vi "detection.vi"() -> (0 "Counts":u32=198)   [LabVIEW 2012]
uses:
  <vilib>/DAQmx/write.llb/DAQmx Write (Digital Wfm 1Chan NSamp).vi
  <vilib>/DAQmx/write.llb/DAQmx Write (Digital 1D Bool 1Chan 1Samp).vi
  <vilib>/DAQmx/read.llb/DAQmx Read (Counter 1D U32 1Chan NSamp).vi
  <vilib>/Waveform/DWDTOps.llb/DWDT Boolean Array to Digital.vi
  <vilib>/DAQmx/create/channels.llb/DAQmx Create Channel (CO-Pulse Generation-Frequency).vi
  <vilib>/DAQmx/configure/timing.llb/DAQmx Timing (Implicit).vi
  <vilib>/DAQmx/create/channels.llb/DAQmx Create Channel (CI-Count Edges).vi
  <vilib>/DAQmx/configure/timing.llb/DAQmx Timing (Sample Clock).vi
  <vilib>/DAQmx/create/channels.llb/DAQmx Create Channel (DO-Digital Output).vi
  <vilib>/Waveform/DWDTOps.llb/DWDT Uncompress Digital.vi
  <vilib>/DAQmx/miscellaneous.llb/DAQmx Fill In Error Info.vi
  <resource>/objmgr/daqmx.rc
panel:
  in  "Use delay":bool
  in  "Final states":bool[](array[boolean])
  in  "Delay (ms)":dbl
  out "data":u32[](graph)=[0, 0, 1, 0, 1, 0, 2, 0, 2, 4, 2, 2, 0, 2, 0, 0, 2, 1, 2, 1]
  out "Output":bool=TRUE
  in  "Threshold":dbl=200.0
  in  "Detection length (ms)":dbl=20.0 min=1.0
  in  "Off times":i32[](array[numeric])=[0, 0, 0, 0, 0, 0, 0, 0]
  in  "On times":i32[](array[numeric])=[0, 0, 0, 0, 0, 0, 0, 0]
  # "Pockel"
  # "LED"
  # "Tsunami"
  # "RF"
  # "Orange"
  # "Blue"
  # "Red"
  # "Times in 0.1 uS"
  # "Use -1 to never switch"
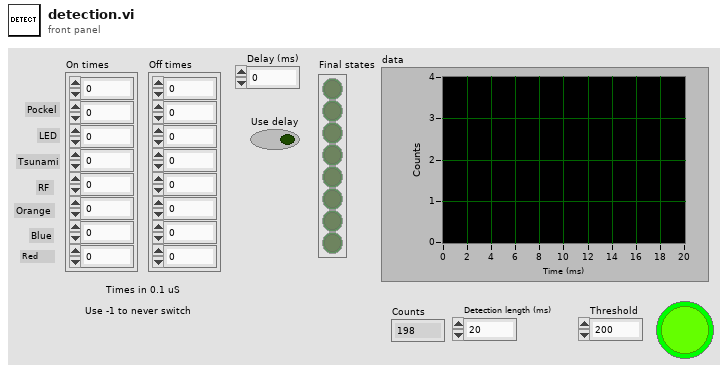
[diagram p1: front panel]
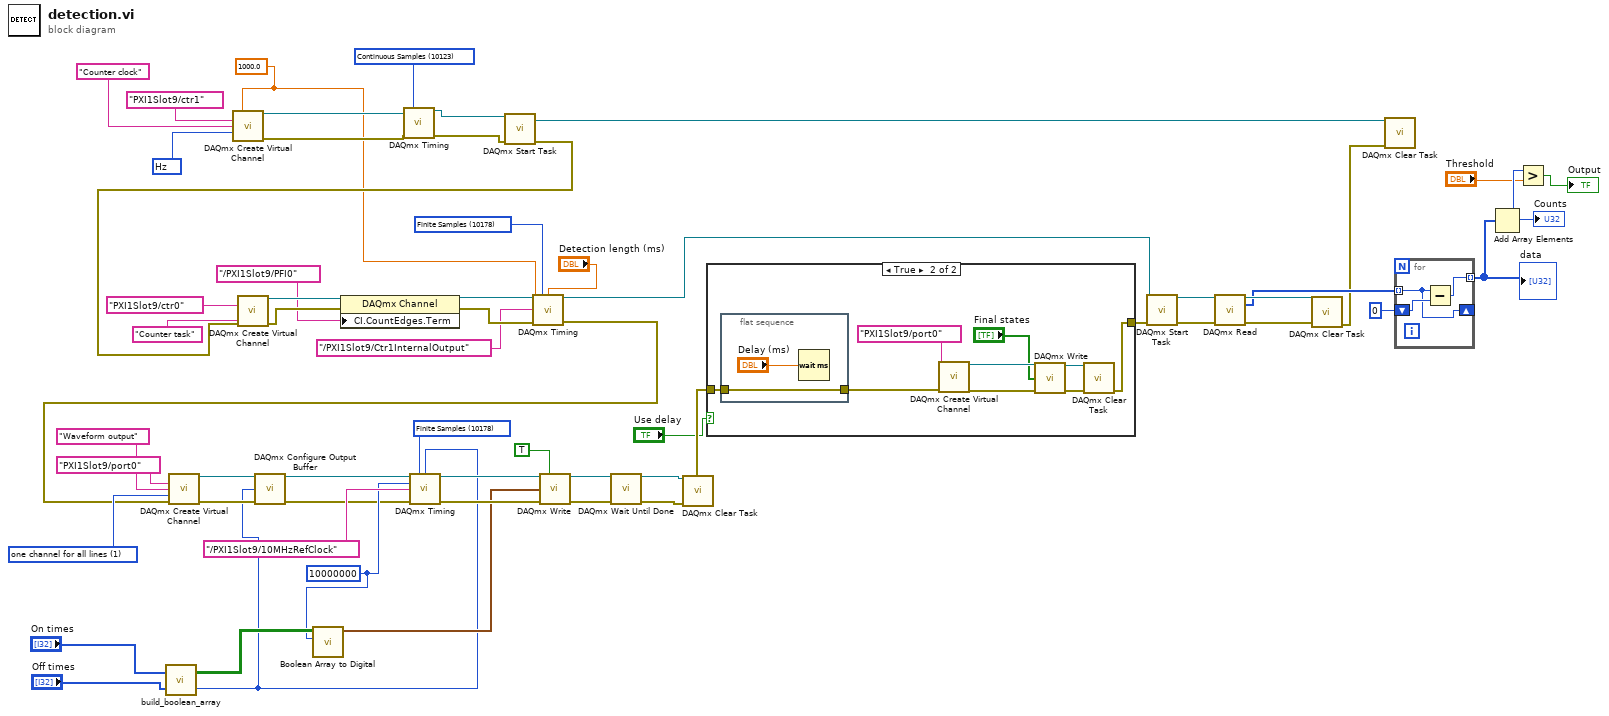
[diagram p0: block diagram]
diagram:
  w29 = 10123 items=["Finite Samples"=10178, "Continuous Samples"=10123, "Hardware Timed Single Point"=12522] ("sample mode")
  w34 = 10373 items=["Hz"=10373] ("units")
  w24 = 1000.0 ("rate")
  w50 = 10178 items=["Finite Samples"=10178, "Continuous Samples"=10123, "Hardware Timed Single Point"=12522] ("sample mode")
  w10 = 10000000 ("rate")
  w57 = 10178 items=["Finite Samples"=10178, "Continuous Samples"=10123, "Hardware Timed Single Point"=12522] ("sample mode")
  w59 = 1 items=["one channel for each line", "one channel for all lines"] ("line grouping")
  n1 = call "build_boolean_array.vi"("Off times"="Off times", "On times"="On times") -> ("max time"=w5:i32, "Array"=w12:bool[][])
  n2 = call-poly <vilib>:"DAQmx Create Virtual Channel.vi"("frequency"=w24, "counter"=tag "PXI1Slot9/ctr1", "name to assign"="Counter clock", "units"=w34) -> ("task out"=w33:refnum<k21>, "error out"=w32:errorcluster)  [unwired: 10 in]
  n3 = call-poly <vilib>:"Boolean Array to Digital.vi"("sample rate"=w10, "boolean array"=w12) -> ("digital waveform"=w11:digitalwaveform)  [unwired: 8 in, 1 out]
  n4 = call-poly <vilib>:"DAQmx Timing.vi"("task/channels in"=w33, "sample mode"=w29, "error in"=w32) -> ("task out"=w31:refnum<k21>, "error out"=w30:errorcluster)  [unwired: 11 in]
  n5 = call <vilib>:"DAQmx Start Task.vi"("task/channels in"=w31, "error in"=w30) -> ("task out"=w26:refnum<k21>, "error out"=w27:errorcluster)  [unwired: 12 in]
  n6 = call-poly <vilib>:"DAQmx Create Virtual Channel.vi"("counter"=tag "PXI1Slot9/ctr0", "name to assign"="Counter task", "error in"=w27) -> ("task out"=w55:refnum<k21>, "error out"=w54:errorcluster)  [unwired: 11 in]
  n7 = property class="DAQmx Channel"(reference=w55, error in=w54, "CI.CountEdges.Term"=tag "/PXI1Slot9/PFI0") -> (reference out=w52:refnum<k21>, error out=w49:errorcluster)
  n8 = call-poly <vilib>:"DAQmx Timing.vi"("task/channels in"=w52, "sample mode"=w50, "samples per channel"="Detection length (ms)", "rate"=w24, "source"=tag "/PXI1Slot9/Ctr1InternalOutput", "error in"=w49) -> ("task out"=w19:refnum<k21>, "error out"=w41:errorcluster)  [unwired: 8 in]
  n9 = call-poly <vilib>:"DAQmx Create Virtual Channel.vi"("lines"=tag "PXI1Slot9/port0", "name to assign"="Waveform output", "line grouping"=w59, "error in"=w41) -> ("task out"=w9:refnum<k21>, "error out"=w7:errorcluster)  [unwired: 10 in]
  n10 = call <vilib>:"DAQmx Configure Output Buffer.vi"("task/channels in"=w9, "buffer size (in samples per channel)"=w5, "error in"=w7) -> ("task out"=w8:refnum<k21>, "error out"=w6:errorcluster)  [unwired: 11 in]
  n11 = call-poly <vilib>:"DAQmx Timing.vi"("task/channels in"=w8, "sample mode"=w57, "samples per channel"=w5, "rate"=w10, "source"=tag "/PXI1Slot9/10MHzRefClock", "error in"=w6) -> ("task out"=w37:refnum<k21>, "error out"=w38:errorcluster)  [unwired: 8 in]
  n12 = call-poly <vilib>:"DAQmx Write.vi"("task/channels in"=w37, "auto start"=TRUE, "data"=w11, "error in"=w38) -> ("task out"=w4:refnum<k21>, "error out"=w3:errorcluster)  [unwired: 9 in, 1 out]
  n13 = call <vilib>:"DAQmx Wait Until Done.vi"("task/channels in"=w4, "error in"=w3) -> ("task out"=w1:refnum<k21>, "error out"=w2:errorcluster)  [unwired: 12 in]
  n14 = call <vilib>:"DAQmx Clear Task.vi"("task in"=w1, "error in"=w2) -> ("error out"=w17:errorcluster)  [unwired: 13 in]
  n15 = case shown="True" "Use delay" {
    tunnel: [w60 w65] -> w18
    tunnel: w17 -> [w60 w61]
    frame False {
    }
    frame True {
      n16 = flat-sequence {
        tunnel: [w70] -> w62
        tunnel: w61 -> [w70]
        frame #0 {
          n17 = Wait (ms)(milliseconds to wait="Delay (ms)") -> ()  [unwired: 1 out]
        }
      }
      n18 = call-poly <vilib>:"DAQmx Create Virtual Channel.vi"("lines"=tag "PXI1Slot9/port0", "error in"=w62) -> ("task out"=w68:refnum<k21>, "error out"=w63:errorcluster)  [unwired: 12 in]
      n19 = call-poly <vilib>:"DAQmx Write.vi"("task/channels in"=w68, "data"="Final states", "error in"=w63) -> ("task out"=w66:refnum<k21>, "error out"=w64:errorcluster)  [unwired: 10 in, 1 out]
      n20 = call <vilib>:"DAQmx Clear Task.vi"("task in"=w66, "error in"=w64) -> ("error out"=w65:errorcluster)  [unwired: 13 in]
    }
  }
  n21 = call <vilib>:"DAQmx Start Task.vi"("task/channels in"=w19, "error in"=w18) -> ("task out"=w39:refnum<k21>, "error out"=w40:errorcluster)  [unwired: 12 in]
  n22 = call-poly <vilib>:"DAQmx Read.vi"("task/channels in"=w39, "error in"=w40) -> ("task out"=w46:refnum<k21>, "data"=w23:u32[], "error out"=w45:errorcluster)  [unwired: 11 in]
  n23 = call <vilib>:"DAQmx Clear Task.vi"("task in"=w46, "error in"=w45) -> ("error out"=w16:errorcluster)  [unwired: 13 in]
  n24 = call <vilib>:"DAQmx Clear Task.vi"("task in"=w26, "error in"=w16) -> ()  [unwired: 13 in, 1 out]
  n25 = for {
    tunnel: w23 -> [w72] mode=indexing
    tunnel: [w73] -> w21 mode=indexing
    shift-right: [w72] -> _
    shift-left: u32 0 ("Numeric") -> [w74]
    n26 = Subtract(x=w72, y=w74) -> (x-y=w73:u32)
  }
  "data" <- w21
  n27 = Add Array Elements(numeric array=w21) -> (sum=w44:u32)
  "Counts" <- w44
  n28 = Greater?(x=w44, y="Threshold") -> (0:→"Output":bool)
